vi "Breakfast Sub vi.vi"() -> (1 "Breakfast Meats":string, 2 "Breakfast Entrees":string, 3 "Breakfast Potato":string, 4 "Breakfast Breads Pastries Toppings":string)   [LabVIEW 2019]
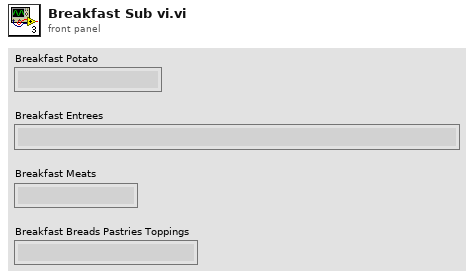
[diagram p1: front panel]
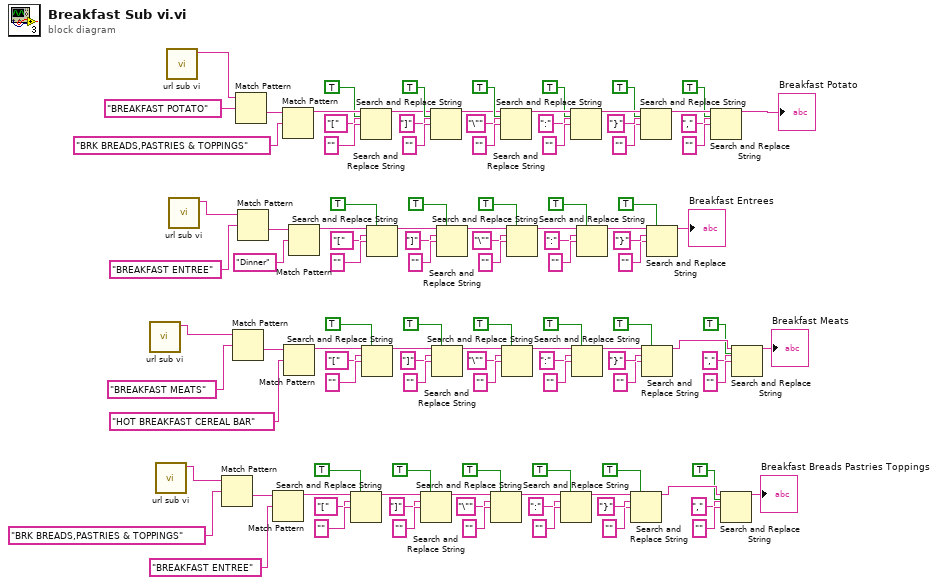
[diagram p0: block diagram]
diagram:
  n1 = call "url sub vi.vi"() -> ("body 2"=w2:string)  [unwired: 11 in]
  n2 = call "url sub vi.vi"() -> ("body 2"=w1:string)  [unwired: 11 in]
  n3 = call "url sub vi.vi"() -> ("body 2"=w4:string)  [unwired: 11 in]
  n4 = call "url sub vi.vi"() -> ("body 2"=w3:string)  [unwired: 11 in]
  n5 = Match Pattern(string=w1, regular expression="BRK BREADS,PASTRIES & TOPPINGS") -> (after substring=w86:string)  [unwired: 1 in, 3 out]
  n6 = Match Pattern(string=w2, regular expression="BREAKFAST MEATS") -> (after substring=w58:string)  [unwired: 1 in, 3 out]
  n7 = Match Pattern(string=w4, regular expression="BREAKFAST POTATO") -> (after substring=w6:string)  [unwired: 1 in, 3 out]
  n8 = Match Pattern(string=w3, regular expression="BREAKFAST ENTREE") -> (after substring=w9:string)  [unwired: 1 in, 3 out]
  n9 = Match Pattern(string=w86, regular expression="BREAKFAST ENTREE") -> (before substring=w88:string)  [unwired: 1 in, 3 out]
  n10 = Match Pattern(string=w6, regular expression="BRK BREADS,PASTRIES & TOPPINGS") -> (before substring=w55:string)  [unwired: 1 in, 3 out]
  n11 = Match Pattern(string=w58, regular expression="HOT BREAKFAST CEREAL BAR") -> (before substring=w60:string)  [unwired: 1 in, 3 out]
  n12 = Match Pattern(string=w9, regular expression="Dinner") -> (before substring=w11:string)  [unwired: 1 in, 3 out]
  n13 = Search and Replace String(replace all?=TRUE ("replace all? (F)"), input string=w88, search string="[", replace string="" ("replace string (\"\")")) -> (result string=w92:string)  [unwired: 4 in, 3 out]
  n14 = Search and Replace String(replace all?=TRUE ("replace all? (F)"), input string=w55, search string="[", replace string="" ("replace string (\"\")")) -> (result string=w39:string)  [unwired: 4 in, 3 out]
  n15 = Search and Replace String(replace all?=TRUE ("replace all? (F)"), input string=w60, search string="[", replace string="" ("replace string (\"\")")) -> (result string=w64:string)  [unwired: 4 in, 3 out]
  n16 = Search and Replace String(replace all?=TRUE ("replace all? (F)"), input string=w11, search string="[", replace string="" ("replace string (\"\")")) -> (result string=w15:string)  [unwired: 4 in, 3 out]
  n17 = Search and Replace String(replace all?=TRUE ("replace all? (F)"), input string=w92, search string="]", replace string="" ("replace string (\"\")")) -> (result string=w96:string)  [unwired: 4 in, 3 out]
  n18 = Search and Replace String(replace all?=TRUE ("replace all? (F)"), input string=w39, search string="]", replace string="" ("replace string (\"\")")) -> (result string=w43:string)  [unwired: 4 in, 3 out]
  n19 = Search and Replace String(replace all?=TRUE ("replace all? (F)"), input string=w64, search string="]", replace string="" ("replace string (\"\")")) -> (result string=w68:string)  [unwired: 4 in, 3 out]
  n20 = Search and Replace String(replace all?=TRUE ("replace all? (F)"), input string=w15, search string="]", replace string="" ("replace string (\"\")")) -> (result string=w19:string)  [unwired: 4 in, 3 out]
  n21 = Search and Replace String(replace all?=TRUE ("replace all? (F)"), input string=w96, search string="\"", replace string="" ("replace string (\"\")")) -> (result string=w102:string)  [unwired: 4 in, 3 out]
  n22 = Search and Replace String(replace all?=TRUE ("replace all? (F)"), input string=w43, search string="\"", replace string="" ("replace string (\"\")")) -> (result string=w49:string)  [unwired: 4 in, 3 out]
  n23 = Search and Replace String(replace all?=TRUE ("replace all? (F)"), input string=w68, search string="\"", replace string="" ("replace string (\"\")")) -> (result string=w74:string)  [unwired: 4 in, 3 out]
  n24 = Search and Replace String(replace all?=TRUE ("replace all? (F)"), input string=w19, search string="\"", replace string="" ("replace string (\"\")")) -> (result string=w25:string)  [unwired: 4 in, 3 out]
  n25 = Search and Replace String(replace all?=TRUE ("replace all? (F)"), input string=w102, search string=":", replace string="" ("replace string (\"\")")) -> (result string=w106:string)  [unwired: 4 in, 3 out]
  n26 = Search and Replace String(replace all?=TRUE ("replace all? (F)"), input string=w49, search string=":", replace string="" ("replace string (\"\")")) -> (result string=w53:string)  [unwired: 4 in, 3 out]
  n27 = Search and Replace String(replace all?=TRUE ("replace all? (F)"), input string=w74, search string=":", replace string="" ("replace string (\"\")")) -> (result string=w78:string)  [unwired: 4 in, 3 out]
  n28 = Search and Replace String(replace all?=TRUE ("replace all? (F)"), input string=w25, search string=":", replace string="" ("replace string (\"\")")) -> (result string=w29:string)  [unwired: 4 in, 3 out]
  n29 = Search and Replace String(replace all?=TRUE ("replace all? (F)"), input string=w106, search string="}", replace string="" ("replace string (\"\")")) -> (result string=w111:string)  [unwired: 4 in, 3 out]
  n30 = Search and Replace String(replace all?=TRUE ("replace all? (F)"), input string=w53, search string="}", replace string="" ("replace string (\"\")")) -> (result string=w56:string)  [unwired: 4 in, 3 out]
  n31 = Search and Replace String(replace all?=TRUE ("replace all? (F)"), input string=w78, search string="}", replace string="" ("replace string (\"\")")) -> (result string=w83:string)  [unwired: 4 in, 3 out]
  n32 = Search and Replace String(replace all?=TRUE ("replace all? (F)"), input string=w29, search string="}", replace string="" ("replace string (\"\")")) -> (result string=→"Breakfast Entrees":string)  [unwired: 4 in, 3 out]
  n33 = Search and Replace String(replace all?=TRUE ("replace all? (F)"), input string=w56, search string=",", replace string="" ("replace string (\"\")")) -> (result string=→"Breakfast Potato":string)  [unwired: 4 in, 3 out]
  n34 = Search and Replace String(replace all?=TRUE ("replace all? (F)"), input string=w111, search string=",", replace string="" ("replace string (\"\")")) -> (result string=→"Breakfast Breads Pastries Toppings":string)  [unwired: 4 in, 3 out]
  n35 = Search and Replace String(replace all?=TRUE ("replace all? (F)"), input string=w83, search string=",", replace string="" ("replace string (\"\")")) -> (result string=→"Breakfast Meats":string)  [unwired: 4 in, 3 out]
